vi "Get LV Class Members from Path.vi"(6 "Shallow (FALSE)":bool, 7 "application reference (local)":refnum<vi>, 8 "error in (no error)":errorcluster, 11 "Class Path":path) -> (0 "error out":errorcluster, 2 "LV Class Members":path[](array[path]))   [LabVIEW 2011, in "VITesterUtilities.lvlib"]
uses:
  Libraries/VITesterUtilities.lvlib
  <userlib>/_OpenG.lib/array/array.llb/Filter 1D Array with Scalar (Path)__ogtk.vi
panel:
  # "Copyright © 2007 James Kring, Inc. All rights reserved.\n\nAuthor: Jim Kring [jim.kring@jameskring.com]\n\nThis library is provided \"AS IS\" ,WITHOUT WARRANTIES OR \nCONDITIONS OF ANY KIND, either express or implied.\n\nJames Kring, Inc. -- http://www.jameskring.com"
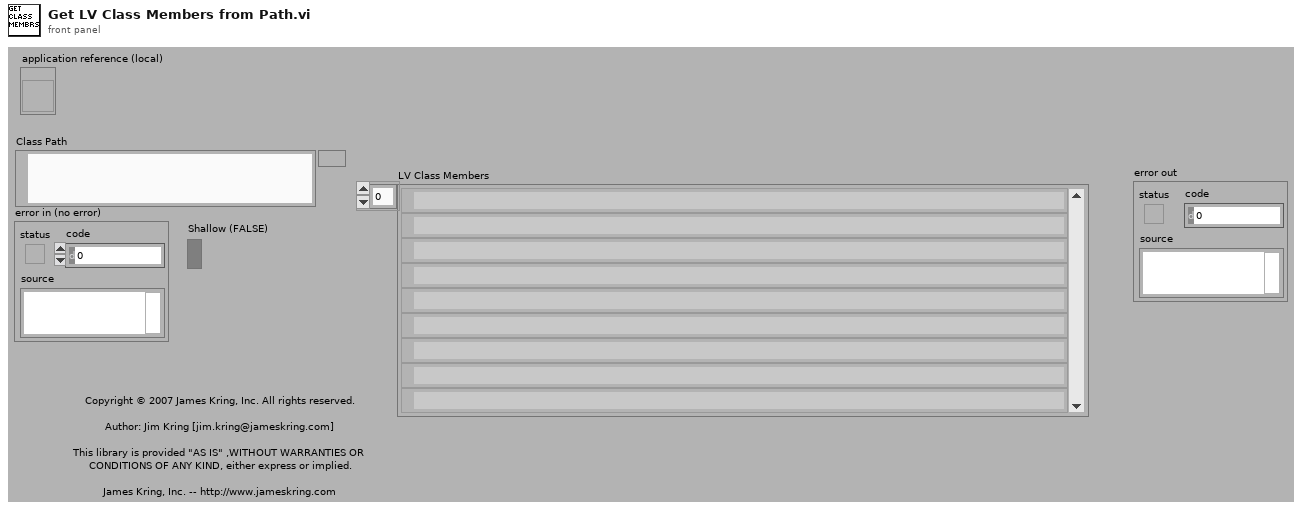
[diagram p1: front panel]
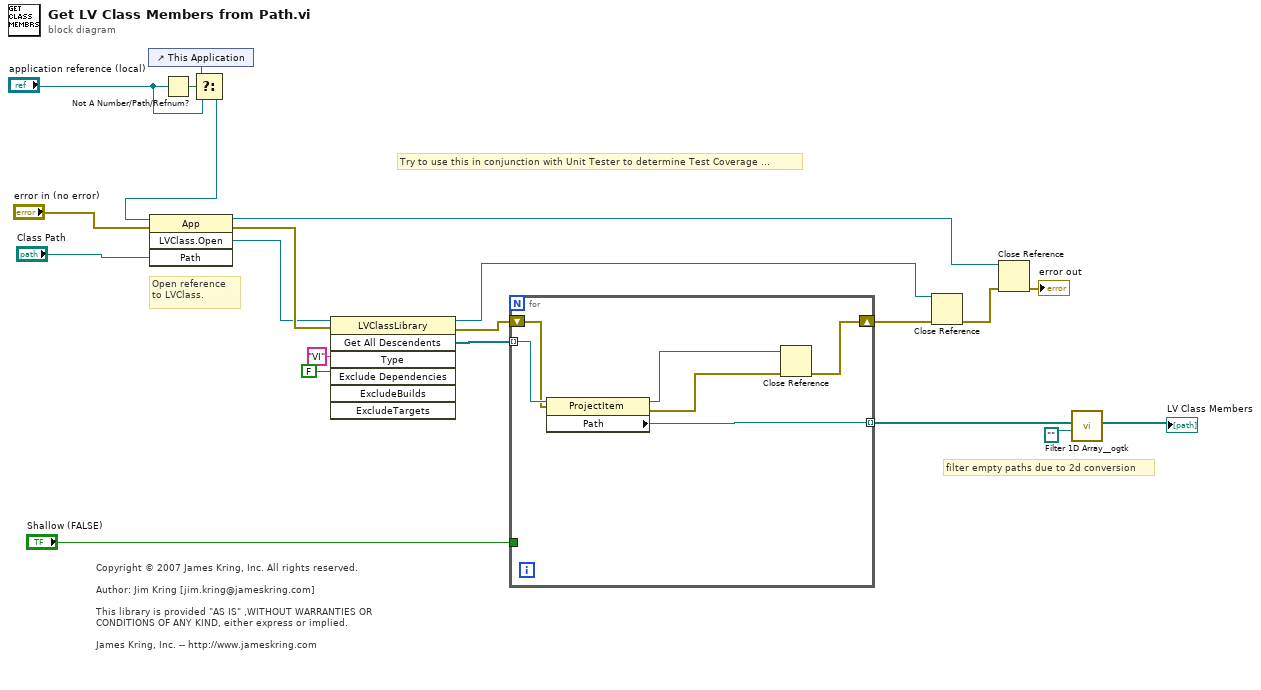
[diagram p0: block diagram]
diagram:
  # "Copyright © 2007 James Kring, Inc. All rights reserved.\n\nAuthor: Jim Kring [jim.kring@jameskring.com]\n\nThis library is provided \"AS IS\" ,WITHOUT WARRANTIES OR \nCONDITIONS OF ANY KIND, either express or implied.\n\nJames Kring, Inc. -- http://www.jameskring.com"
  # "filter empty paths due to 2d conversion"
  # "Try to use this in conjunction with Unit Tester to determine Test Coverage ..."
  # "Open reference to LVClass."
  n1 = control-ref of="This Application"() -> (w5:refnum<vi>)
  n2 = Not A Number/Path/Refnum?(number/path/refnum="application reference (local)") -> (NaN/Path/Refnum?=w4:bool)
  n3 = Select(t=w5, s=w4, f="application reference (local)") -> (s? t:f=w2:refnum<vi>)
  n4 = invoke class="App" method="LVClass.Open"(reference=w2, error in="error in (no error)", "Path"="Class Path") -> (reference out=w7:refnum<vi>, error out=w17:errorcluster, "LVClass.Open"=w10:refnum<vi>)  [unwired: 1 in, 1 out]
  n5 = invoke class="LVClassLibrary" method="Get All Descendents"(reference=w10, error in=w17, "Type"="VI", "Exclude Dependencies"=FALSE ("ExcludeDependencies")) -> (reference out=w11:refnum<vi>, error out=w16:errorcluster, "All Descendents"=w19:refnum<vi>[])  [unwired: 3 in, 4 out]
  n6 = for {
    tunnel: w19 -> [w26] mode=indexing
    shift-right: [w24] -> w15
    shift-left: w16 -> [w25]
    tunnel: [w23] -> w12 mode=indexing
    tunnel: "Shallow (FALSE)" -> [_]
    n7 = property class="ProjectItem"(reference=w26, error in=w25) -> (reference out=w27:refnum<vi>, error out=w22:errorcluster, "Path"=w23:path)
    n8 = Close Reference(reference=w27, error in (no error)=w22) -> (error out=w24:errorcluster)
  }
  n9 = Close Reference(reference=w11, error in (no error)=w15) -> (error out=w18:errorcluster)
  n10 = Close Reference(reference=w7, error in (no error)=w18) -> (error out=→"error out":errorcluster)
  n11 = call-poly <userlib>:"Filter 1D Array__ogtk.vi"("items to filter"=path "", "array"=w12) -> ("filtered array"=→"LV Class Members":path[])  [unwired: 4 in, 1 out]
